vi "Strip Quotes.vi"(8 "error in (no error)":errorcluster, 11 "String":string) -> (0 "error out":errorcluster, 3 "result string":string)   [LabVIEW 2011, in "JSON Value.lvclass"]
uses:
  JSON Value/JSON Value.lvclass
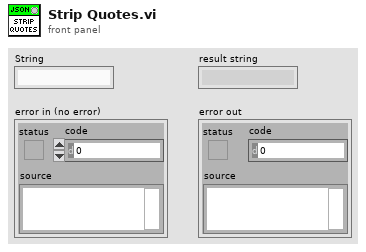
[diagram p1: front panel]
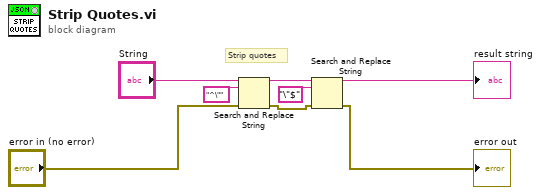
[diagram p0: block diagram]
diagram:
  # "Strip quotes"
  n1 = Search and Replace String(input string="String", search string="^\"", error in="error in (no error)") -> (result string=w4:string, error out=w7:errorcluster)  [unwired: 5 in, 2 out]
  n2 = Search and Replace String(input string=w4, search string="\"$", error in=w7) -> (result string=→"result string":string, error out=→"error out":errorcluster)  [unwired: 5 in, 2 out]
